vi "InitHardware.vi"(8 "error in (no error)":errorcluster, 11 "PCO in":refnum<class "PCO_Camera.lvclass">) -> (0 "error out":errorcluster, 1 "bit depth":string, 2 "Image Type":T3 items=["Grayscale (U8)", "Grayscale (I16)", "Grayscale (SGL)", "Complex (CSG)", "RGB (U32)", "HSL (U32)", "RGB (U64)", "Grayscale (U16)"], 3 "PCO out":refnum<class "PCO_Camera.lvclass">)   [LabVIEW 2020, in "PCO_Camera.lvclass"]
uses:
  PCO_Camera.lvclass
  C:/GEECS/Developers Version/source/Device Drivers/Point Grey Camera/Point Grey Camera.lvclass
  pco.labview/pco.camera/Controls/binning.ctl
  Point Grey Camera/Point Grey Camera.lvclass/Point Grey Camera.ctl
  PCO_Camera.lvclass/PCO_Camera.ctl
  Point Grey Camera/Read Settings 2.vi
  Point Grey Camera/Write Settings 2.vi
  pco.labview/pco.camera/Camera.lvclass
panel:
  out "max_height":u64
  out "max_width":u64
  out "Info Post Init":T2
  out "Info Pre Inti":T2
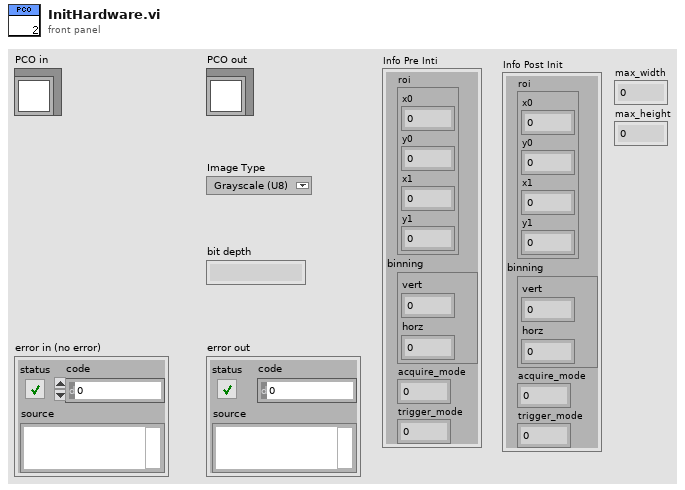
[diagram p1: front panel]
types:
  T1 = typedef "Camera.lvclass/binning.ctl" = cluster{"vert":u16, "horz":u16}
  T2 = cluster{"roi":cluster{"x0":u64, "y0":u64, "x1":u64, "y1":u64}, "binning":T1, "acquire_mode":u16, "trigger_mode":u16}
  T3 = typedef "Image Type" = u32
  T4 = enum16{"sequence", "sequence non blocking", "ring buffer", "fifo", "sequence_dpcore", "sequence_non_blocking_dpcore", "ring_buffer_dpcore", "fifo_dpcore", "tif", "multitif", "pcoraw", "b16", "dicom", "multidicom"}
  T5 = typedef "Point Grey Camera.lvclass/SettingsTypdef.ctl" = cluster{"Trigger":T6, "Gain":cluster{"Value":dbl, "Min":dbl, "Max":dbl, "StepSize":dbl, "Tolerance":dbl, "valueactual":dbl}, "Exposure":cluster{"Value":dbl, "Min":dbl, "Max":dbl, "StepSize":dbl, "Tolerance":dbl, "valueactual":dbl}, "Timeout":cluster{"Value":dbl, "Min":dbl, "Max":dbl, "StepSize":dbl, "Tolerance":dbl, "valueactual":dbl}, "LocalSavingPath":path, "Save":T6, "TriggerDelay":cluster{"Value":dbl, "Min":dbl, "Max":dbl, "StepSize":dbl, "Tolerance":dbl, "valueactual":dbl}, "CamSession":string, "ROI":T7, "MaxGUIPixel":cluster{"Value":dbl, "Min":dbl, "Max":dbl, "StepSize":dbl, "Tolerance":dbl, "valueactual":dbl}, "Target":cluster{"X":cluster{"Value":dbl, "Min":dbl, "Max":dbl, "StepSize":dbl, "Tolerance":dbl, "valueactual":dbl}, "Y":cluster{"Value":dbl, "Min":dbl, "Max":dbl, "StepSize":dbl, "Tolerance":dbl, "valueactual":dbl}}, "Analysis":T6, "maxshot#":dbl, "SpatialCalibration":cluster{"Value":dbl, "Min":dbl, "Max":dbl, "StepSize":dbl, "Tolerance":dbl, "valueactual":dbl}, "roistatus":T6, "Lineout":T6, "AnalysisThreshold":cluster{"Value":dbl, "Min":dbl, "Max":dbl, "StepSize":dbl, "Tolerance":dbl, "valueactual":dbl}, "TargetSize":cluster{"X":cluster{"Value":dbl, "Min":dbl, "Max":dbl, "StepSize":dbl, "Tolerance":dbl, "valueactual":dbl}, "Y":cluster{"Value":dbl, "Min":dbl, "Max":dbl, "StepSize":dbl, "Tolerance":dbl, "valueactual":dbl}}, "Simulation":T6, "SpatialCalibrationY":cluster{"Value":dbl, "Min":dbl, "Max":dbl, "StepSize":dbl, "Tolerance":dbl, "valueactual":dbl}, "Target2":cluster{"X":cluster{"Value":dbl, "Min":dbl, "Max":dbl, "StepSize":dbl, "Tolerance":dbl, "valueactual":dbl}, "Y":cluster{"Value":dbl, "Min":dbl, "Max":dbl, "StepSize":dbl, "Tolerance":dbl, "valueactual":dbl}}, "Target2Size":cluster{"X":cluster{"Value":dbl, "Min":dbl, "Max":dbl, "StepSize":dbl, "Tolerance":dbl, "valueactual":dbl}, "Y":cluster{"Value":dbl, "Min":dbl, "Max":dbl, "StepSize":dbl, "Tolerance":dbl, "valueactual":dbl}}, "Crosshair":cluster{"Label1":string, "Label2":string}, "Max2ndMomRadius":cluster{"Value":dbl, "Min":dbl, "Max":dbl, "StepSize":dbl, "Tolerance":dbl, "valueactual":dbl}, "SaveType":T8, "BackgroundPath":path, "GUI8bit":T6, "GUICompression":T6, "CompressionQuality":cluster{"Value":dbl, "Min":dbl, "Max":dbl, "StepSize":dbl, "Tolerance":dbl, "valueactual":dbl}, "SaveAsync":T6, "PerspectivePath":path, "PerspectiveCorrectGUI":T6, "BlackLevel":cluster{"Value":dbl, "Min":dbl, "Max":dbl, "StepSize":dbl, "Tolerance":dbl, "valueactual":dbl}, "TargetBP":cluster{"X":cluster{"Value":dbl, "Min":dbl, "Max":dbl, "StepSize":dbl, "Tolerance":dbl, "valueactual":dbl}, "Y":cluster{"Value":dbl, "Min":dbl, "Max":dbl, "StepSize":dbl, "Tolerance":dbl, "valueactual":dbl}}, "PythonAnalysis":T6, "PythonFunctionName":string, "PythonLineout":T6, "PythonVersion":string, "GEECSBuildsPath":path, "DisplayPythonProcessedImage":T6, "PythonModuleName":string, "AnalysisThresholdHigh":cluster{"Value":dbl, "Min":dbl, "Max":dbl, "StepSize":dbl, "Tolerance":dbl, "valueactual":dbl}, "AnalysisMedianRank":cluster{"Value":dbl, "Min":dbl, "Max":dbl, "StepSize":dbl, "Tolerance":dbl, "valueactual":dbl}, "ClockSpeed":cluster{"Value":dbl, "Min":dbl, "Max":dbl, "StepSize":dbl, "Tolerance":dbl, "valueactual":dbl}, "AutoTrigger":T6, "AutoTriggerLevelMeanCounts":cluster{"Value":dbl, "Min":dbl, "Max":dbl, "StepSize":dbl, "Tolerance":dbl, "valueactual":dbl}, "AnalysisROILeft":cluster{"Value":dbl, "Min":dbl, "Max":dbl, "StepSize":dbl, "Tolerance":dbl, "valueactual":dbl}, "AnalysisROIRight":cluster{"Value":dbl, "Min":dbl, "Max":dbl, "StepSize":dbl, "Tolerance":dbl, "valueactual":dbl}, "AnalysisROITop":cluster{"Value":dbl, "Min":dbl, "Max":dbl, "StepSize":dbl, "Tolerance":dbl, "valueactual":dbl}, "AnalysisROIBottom":cluster{"Value":dbl, "Min":dbl, "Max":dbl, "StepSize":dbl, "Tolerance":dbl, "valueactual":dbl}, "AnalysisROI":T6, "UseSoftwareTrigger":T6, "UDPtrigger":T6, "AutoTriggerLevelMaxCounts":cluster{"Value":dbl, "Min":dbl, "Max":dbl, "StepSize":dbl, "Tolerance":dbl, "valueactual":dbl}}
  T6 = typedef "OnOffTypeDef.ctl" = enum16{"off", "on"}
  T7 = typedef "ROI_TypDef.ctl" = cluster{"Width":cluster{"Value":dbl, "Min":dbl, "Max":dbl, "StepSize":dbl, "Tolerance":dbl, "valueactual":dbl}, "Height":cluster{"Value":dbl, "Min":dbl, "Max":dbl, "StepSize":dbl, "Tolerance":dbl, "valueactual":dbl}, "OffsetX":cluster{"Value":dbl, "Min":dbl, "Max":dbl, "StepSize":dbl, "Tolerance":dbl, "valueactual":dbl}, "OffsetY":cluster{"Value":dbl, "Min":dbl, "Max":dbl, "StepSize":dbl, "Tolerance":dbl, "valueactual":dbl}}
  T8 = typedef "Image save type.ctl" = enum16{"PNG", "BMP", "JPEG", "TDMS", "hdf5"}
  T9 = cluster{"serial":u32, "type":u16, "sub_type":u16, "interface_type":u16, "bit_resolution":u16, "min_exposure_time_s":dbl, "max_exposure_time_s":dbl, "min_exposure_step_s":dbl, "min_delay_time_s":dbl, "max_delay_time_s":dbl, "min_delay_step_s":dbl, "min_width":u64, "min_height":u64, "max_width":u64, "max_height":u64, "roi_step_horz":u64, "roi_step_vert":u64, "roi_symmetric_horz":bool, "roi_symmetric_vert":bool, "has_timestamp_mode":bool, "has_timestamp_mode_ascii_only":bool, "pixelrate_vec":u32[], "has_acquire_mode":bool, "has_ext_acquire_mode":bool, "has_metadata_mode":bool, "has_ram":bool, "binning_horz_vec":u16[], "binning_vert_vec":u16[]}
  T10 = cluster{"exposure_time_s":dbl, "delay_time_s":dbl, "roi":cluster{"x0":u64, "y0":u64, "x1":u64, "y1":u64}, "timestamp_mode":u16, "pixelrate":u32, "trigger_mode":u16, "acquire_mode":u16, "metadata_mode":u16, "noisefilter_mode":u16, "binning":T1}
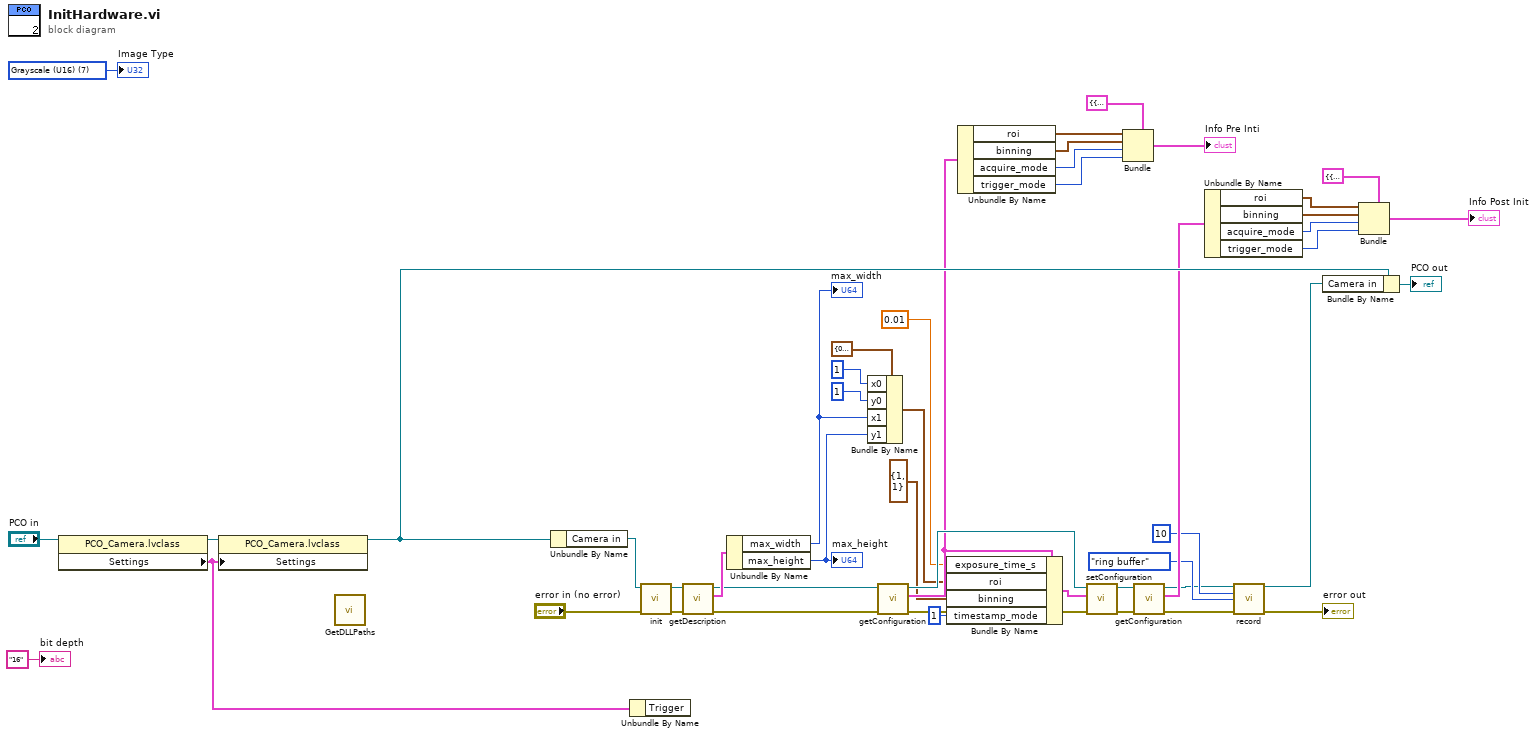
[diagram p0: block diagram]
diagram:
  w44 = T3 7 items=["Grayscale (U8)", "Grayscale (I16)", "Grayscale (SGL)", "Complex (CSG)", "RGB (U32)", "HSL (U32)", "RGB (U64)", "Grayscale (U16)"] ("Image Type")
  n1 = property class="PCO_Camera.lvclass"(reference="PCO in") -> (reference out=w43:refnum<class "PCO_Camera.lvclass">, "Settings"=w2:T5)  [unwired: 1 in, 1 out]
  n2 = property class="PCO_Camera.lvclass"(reference=w43, "Settings"=w2) -> (reference out=w34:refnum<class "PCO_Camera.lvclass">)  [unwired: 1 in, 1 out]
  n3 = call "GetDLLPaths.vi"() -> ()  [unwired: 9 in, 3 out]
  n4 = Unbundle By Name(w34) -> ("Camera in"=w1:refnum<class "Camera.lvclass">)
  n5 = Unbundle By Name(w2) -> ()  [unwired: 1 out]
  n6 = call-dynamic "init.vi"("Camera in"=w1, "error in (no error)"="error in (no error)") -> ("Camera out"=w42:refnum<class "Camera.lvclass">, "error out"=w21:errorcluster)  [unwired: 7 in]
  n7 = call-dynamic "getDescription.vi"("error in (no error)"=w21, "Camera in"=w42) -> ("error out"=w20:errorcluster, "description"=w41:T9, "Camera out"=w33:refnum<class "Camera.lvclass">)  [unwired: 7 in]
  n8 = Unbundle By Name(w41) -> ("max_width"=w25:u64, "max_height"=w24:u64)
  "max_width" <- w25
  "max_height" <- w24
  n9 = Bundle By Name(cluster=cluster{"x0":u64, "y0":u64, "x1":u64, "y1":u64} {"x0"=0, "y0"=0, "x1"=0, "y1"=0} ("roi"), "x0"=u64 1, "y0"=u64 1, "x1"=w25, "y1"=w24) -> (w23:cluster{"x0":u64, "y0":u64, "x1":u64, "y1":u64})
  n10 = call-dynamic "getConfiguration.vi"("error in (no error)"=w20, "Camera in"=w33) -> ("error out"=w19:errorcluster, "configuration"=w31:T10, "Camera out"=w32:refnum<class "Camera.lvclass">)  [unwired: 7 in]
  n11 = Bundle By Name(cluster=w31, "exposure_time_s"=0.01, "roi"=w23, "binning"=T1 {"vert"=1, "horz"=1}, "timestamp_mode"=u16 1 ("metadata_mode")) -> (w30:T10)
  n12 = Unbundle By Name(w31) -> ("roi"=w40:cluster{"x0":u64, "y0":u64, "x1":u64, "y1":u64}, "binning"=w39:T1, "acquire_mode"=w38:u16, "trigger_mode"=w37:u16)
  n13 = call-dynamic "setConfiguration.vi"("error in (no error)"=w19, "configuration"=w30, "Camera in"=w32) -> ("error out"=w15:errorcluster, "Camera out"=w16:refnum<class "Camera.lvclass">)  [unwired: 7 in]
  n14 = Bundle(cluster=T2 {"roi"={"x0"=0, "y0"=0, "x1"=0, "y1"=0}, "binning"={"vert"=0, "horz"=0}, "acquire_mode"=0, "trigger_mode"=0} ("output cluster"), "roi"=w40, "binning"=w39, "acquire_mode"=w38, "trigger_mode"=w37) -> (→"Info Pre Inti":T2)
  n15 = call-dynamic "getConfiguration.vi"("error in (no error)"=w15, "Camera in"=w16) -> ("error out"=w5:errorcluster, "configuration"=w14:T10, "Camera out"=w7:refnum<class "Camera.lvclass">)  [unwired: 7 in]
  n16 = Unbundle By Name(w14) -> ("roi"=w13:cluster{"x0":u64, "y0":u64, "x1":u64, "y1":u64}, "binning"=w12:T1, "acquire_mode"=w11:u16, "trigger_mode"=w10:u16)
  n17 = call-dynamic "record.vi"("Camera in"=w7, "num_images"=u32 10, "record_mode"=T4."ring buffer", "error in (no error)"=w5) -> ("Camera out"=w6:refnum<class "Camera.lvclass">, "error out"=→"error out":errorcluster)  [unwired: 10 in]
  n18 = Bundle By Name(cluster=w34, "Camera in"=w6) -> (→"PCO out":refnum<class "PCO_Camera.lvclass">)
  n19 = Bundle(cluster=T2 {"roi"={"x0"=0, "y0"=0, "x1"=0, "y1"=0}, "binning"={"vert"=0, "horz"=0}, "acquire_mode"=0, "trigger_mode"=0} ("output cluster"), "roi"=w13, "binning"=w12, "acquire_mode"=w11, "trigger_mode"=w10) -> (→"Info Post Init":T2)
  "Image Type" <- w44
  "bit depth" <- "16" ("bit depth")
